vi "TestTemplate.vi"() -> ()   [LabVIEW 2016, in "TestLibrary.lvlib"]
doc: "Contain the test template for creating test cases"
uses:
  TestLibrary.lvlib
  <vilib>/SLL Drona/APIs/Stimulus/ControlValue/SetValueAuto.vi
  <vilib>/SLL Drona/APIs/Assert/AssertControlValue/Equal.vi
  <vilib>/SLL Drona/Drona.lvlib
  <vilib>/SLL Drona/APIs/Stimulus/ControlValue/ControlValue.lvlib
  <vilib>/SLL Drona/APIs/Assert/AssertControlValue/AssertControlValue.lvlib
panel:
  out "error out":errorcluster
  in  "error in (no error)":errorcluster
  # "Test Template"
  # "Note:  All the testcase names should start \nwith prefix \"Test\""
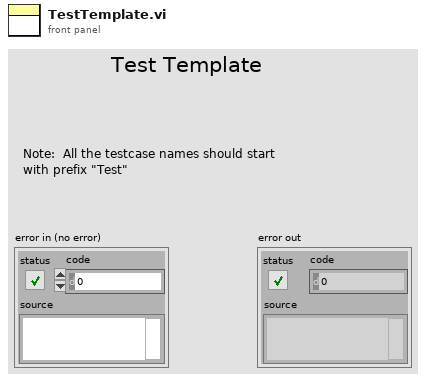
[diagram p1: front panel]
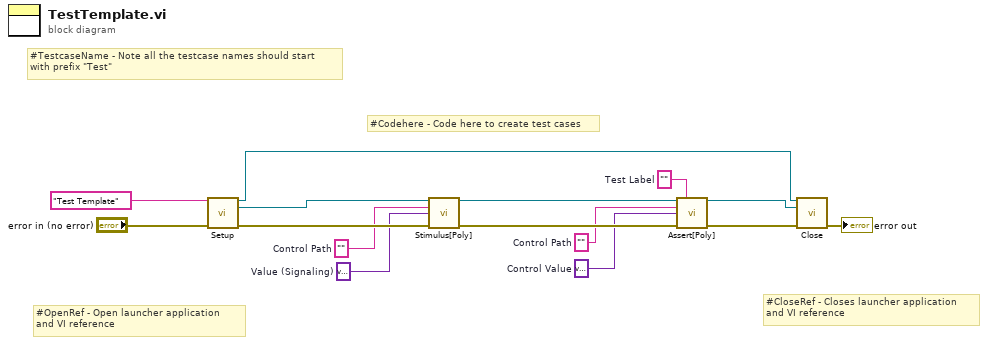
[diagram p0: block diagram]
diagram:
  w3 = ""  # Test Label
  w4 = variant  # Control Value
  w5 = ""  # Control Path
  w6 = variant  # Value (Signaling)
  w7 = ""  # Control Path
  # "#CloseRef - Closes launcher application\nand VI reference"
  # "#OpenRef - Open launcher application\nand VI reference"
  # "#Codehere - Code here to create test cases"
  # "#TestcaseName - Note all the testcase names should start \nwith prefix \"Test\""
  n1 = call <vilib>:"Setup.vi"("Test Label"="Test Template", "error in"="error in (no error)") -> ("Application Ref"=w11:refnum<vi>, "VI Reference Out"=w10:refnum<vi>, "error out"=w14:errorcluster)  [unwired: 11 in]
  n2 = call-poly <vilib>:"Stimulus[Poly].vi"("VI Reference In"=w10, "Control Path"=w7, "Value (Signaling)"=w6, "error in"=w14) -> ("VI Reference Out"=w9:refnum<vi>, "error out"=w13:errorcluster)  [unwired: 10 in]
  n3 = call-poly <vilib>:"Assert[Poly].vi"("VI Reference In"=w9, "Test Label"=w3, "Control Path"=w5, "Control Value"=w4, "Error In"=w13) -> ("VI Reference Out"=w8:refnum<vi>, "Error Out"=w12:errorcluster)  [unwired: 8 in, 1 out]
  n4 = call <vilib>:"Close.vi"("Application Ref"=w11, "VI Reference"=w8, "error in"=w12) -> ("error out"=→"error out":errorcluster)  [unwired: 12 in]
